vi "sub_load-val.vi"(7 "cmd":enum16{"load", "save"}(ring), 8 "Error in":errorcluster) -> (0 "error out":errorcluster caption="Error out", 3 "config 2":T1={"Ch"="cDAQ1Mod1/ao0", "Max V"=5.0, "Min V"=-5.0, " Rate"=1000.0, "N pts"=100, "sample mode"=10178} {"sample mode" items=["유한 샘플"=10178, "연속 샘플"=10123, "하드웨어 타이밍에 의한 단일 포인트"=12522]})   [LabVIEW 2019]
uses:
  _ctrl/cDAQ-9269 Config.ctl
  _ctrl/TestType.ctl
  _ctrl/rw.ctl
  _ctrl/DL950_config.ctl
  _ctrl/BP4610_config.ctl
  _ctrl/DSP_config.ctl
  Devices/NI Board/cDAQ-9221 AI/Set_NIAI.ctl
  Devices/NI Board/cDAQ-9269 AO/Set_AO_Wave-config.ctl
  Global_params.vi
  Capacitor/Global_params_cap.vi
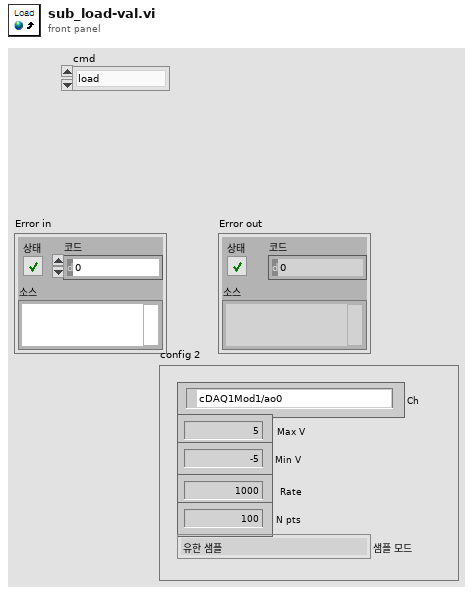
[diagram p1: front panel]
types:
  T1 = typedef "cDAQ-9269 Config.ctl" = cluster{"Ch":tag, "Max V":dbl, "Min V":dbl, " Rate":dbl, "N pts":i32, "sample mode":i32}
  T2 = typedef "TestType.ctl" = enum16{"Manual", "Reg", "Cap", "B1", "B2", "B3"}
  T3 = typedef "rw.ctl" = enum16{"read", "write"}
  T4 = typedef "DL950_config.ctl" = cluster{"Timeout":u32, "Time Div":i32, "Acq Mode":i32, "Record Len":i32, "Record Num":i32, "Start Point":i64, "End Poin":i64, "Visa":refnum<visa-resource-name>, "Config Voltage":cluster{"Enable":bool, "Ch":u16, "V Div":i32, "Coupling":i32, "Probe":i32, "Act.Items":bool, "items":i32[]}[], "Trigger on":bool, "Trigger Level":dbl, "Reset":bool, "Config Temp":cluster{"Channel":u16, "Burn Out":bool, " Type ":i32}[], "Trig Mode":i32, "Trig Pos":dbl, "Trigger Slope":i32, "Trigger Source ":i32, "Trig Start -5":dbl, "End 5":dbl}
  T5 = cluster{"Enable":bool, "Ch":u16, "V Div":i32, "Coupling":i32, "Probe":i32, "Act.Items":bool, "items":i32[]}[]
  T6 = typedef "BP4610_config.ctl" = cluster{"VISA":refnum<visa-resource-name>, "Limit-BP":cluster{"Set":enum16{"Current", "Voltage"}, "Voltage+[V]":dbl, "Current+[A]":dbl, "Voltage-[V]":dbl, "Current-[A]":dbl}, "SET BP":cluster{"Set":enum16{"Current", "Voltage", "FREQ/WAVE"}, "Operation mode":u16, "Voltage[Vp-p]":dbl, "Current[Ap-p]":dbl, "Voltage[V]":dbl, "Current[A]":dbl, "Frequency[Hz]":dbl, "Waveform":enum16{"Sine", "Square", "ARB 1", "ARB 2", "ARB 3", "ARB 4", "ARB 5", "ARB 6", "ARB 7", "ARB 8", "ARB 9", "ARB 10", "ARB 11", "ARB 12", "ARB 13", "ARB 14", "ARB 15", "ARB 16"}}}
  T7 = cluster{"Set":enum16{"Current", "Voltage"}, "Voltage+[V]":dbl, "Current+[A]":dbl, "Voltage-[V]":dbl, "Current-[A]":dbl}
  T8 = typedef "DSP_config.ctl" = cluster{"Port":refnum<visa-resource-name>, "OVP Level":dbl, "OCP Level":dbl, "Current":dbl, "Voltage":dbl}
  T9 = typedef "Set_NIAI.ctl" = cluster{"input terminal":i32, "minimum value":dbl, "maximum value":dbl, "number of samples":i32, "rate":dbl, "sample mode":i32, "physical channels":tag}
  T10 = typedef "Set_AO_Wave-config.ctl" = cluster{"offset":dbl, "Samples":i32, "duty":dbl, "Rate":dbl, "wfm":cluster{"Freq":dbl, "Amp":dbl, "Type":enum16{"Sine Wave", "Triangle Wave", "Square Wave", "Sawtooth Wave"}}}
  T11 = typedef "ref_all.ctl" = cluster{"BP4610 Config":refnum<vi>, "DSP1950 Config":refnum<vi>, "2470-config":refnum<vi>, "cDAQ 9269 AO config":refnum<vi>, "cDAQ 9221 Config":refnum<vi>, "cDAQ-9467 Config":refnum<vi>, "Waveform":refnum<vi>, "DL950 wfm":refnum<vi>, "AI Graph":refnum<vi>, "AO_Wave-config":refnum<vi>, "DL950 items":refnum<vi>, "Volt":refnum<vi>, "Current":refnum<vi>, "AO_Level":refnum<vi>, "RC-Test Judgement ":refnum<vi>, "Log path":refnum<vi>, "시험명":refnum<vi>, "file renew[Hr]":refnum<vi>, "Breakdown-Spec":refnum<vi>, "paste":refnum<vi>, "copy":refnum<vi>, "DL950_config":refnum<vi>, "종료시간":refnum<vi>, "경과시간":refnum<vi>, "Apply":refnum<vi>, "DSP Config LV ":refnum<vi>, "Testconfig":refnum<vi>}
  T12 = typedef "Tpye_ParaAll.ctl" = cluster{"DL950_config":T4, "BP4610 Config":T6, "DSP1950 Config":T8, "DMM 2470 Config":cluster{"Source Mode":enum16{"Voltage", "Current"}, "Source Limit Level":dbl, "Source Level":dbl, "Output_2470":bool}, "cDAQ-9221 Config":T9, "cDAQ-9467 Config":tag, "cDAQ-9269 AO Config":T1, "AO_Wave-config":T10, "DSP1950 Config LV":T8}
  T13 = cluster{"Source Mode":enum16{"Voltage", "Current"}, "Source Limit Level":dbl, "Source Level":dbl, "Output_2470":bool}
  T14 = typedef "cap_config.ctl" = cluster{"Test Mode":T15, "ON time[ms]":dbl, "OFF time[ms]":dbl, "1. 작동시간[분]":dbl, "2. 미작동시간[분]":dbl, "3. 작동시간[분]":dbl, "level[V]":dbl, "duty":dbl, "Freq":dbl, "Voltage+[V]":dbl, "Voltage-[V]":dbl, "Current+[A]":dbl, "Current-[A]":dbl, "출력전압[V]":dbl, "출력전류[A]":dbl, "OVP Level":dbl, "OCP Level":dbl, "Time Div":u16, "Record Len":i32, "방전 기준[V]":dbl, "Repeate (Each Ch)":u32, "Cycle[N]":u32, "작동간격[분]":dbl, "TrigPos[%]":dbl, "시험시간[분]":dbl}
  T15 = typedef "시험모드선택.ctl" = enum16{"6.3.1 온도방치 시험", "6.3.2 저온 작동/방치 시험", "6.3.3 고온 작동/방치 시험", "6.3.4 온도 싸이클 시험", "6.3.6 온습도 싸이클 시험", "6.3.7 고온고습 방치", "6.3.8 결로 시험", "6.3.9 빙결시험", "6.3.11.1 작동가진", "6.3.12 충격시험"}
  T16 = typedef "Breakdown-Spec.ctl" = cluster{"제어단 단선 Irms[mA](이하)":dbl, "제어단 특성 전류 Irms[mA] Max":dbl, "제어단 특성 전류 Irms[mA] Min":dbl, "출력단 단선 Irms[mA](이하)":dbl, "출력단 특성 전류 Irms[mA]  Max":dbl, "출력단 특성전류 Irms[mA]  Min":dbl, "온도[degree]":dbl}
  T17 = typedef "Testing-info.ctl" = cluster{"전체채널수":u8, "현재채널번호":u8, "Irms":dbl, "입력전압":dbl, "입력전류":dbl, "출력전압":dbl, "출력전류":dbl, "온도":dbl, "제어단 단선":bool, "제어단 단락":bool, "제어단 특성변화":bool, "출력단 단선":bool, "출력단 단락":bool, "출력단 특성변화":bool, "출력단 전압":bool, "카운트 일치":bool, "Irms 판정":bool, "온도":bool, "테스트 회수":u32, "TestType":T18, "현재회수":u32, "Ch selection":cluster{"1ch":bool, "2ch":bool, "3ch":bool, "4ch":bool, "5ch":bool, "6ch":bool}, "반복":u32, "Path":path, "파일생성주기":u32, "start time":dbl, "stop time":dbl, "현재반복회수":u32, "NG":cluster{"입출력 카운트":bool, "출력전류RMS":bool}}
  T18 = typedef "sequence_single.ctl" = enum16{"Register", "RC", "B1", "B2", "B3", "Oper_LV", "Oper_HV", "ContR_LV"}
  T19 = typedef "cap_params-all.ctl" = cluster{"Basics":cluster{"TestName":string, "Result path":path, "파일 생성 주기[N]":dbl}, "CapTestConfig":T14, "TestSpec":T16}
  T20 = cluster{"DL950_config":T4, "BP4610 Config":T6, "DSP1950 Config":T8, "DMM 2470 Config":cluster{"Source Mode":enum16{"Voltage", "Current"}, "Source Limit Level":dbl, "Source Level":dbl, "Output_2470":bool}, "cDAQ-9221 Config":T9, "cDAQ-9467 Config":tag, "cDAQ-9269 AO Config":T1, "AO_Wave-config":T10, "Cap Params":T19, "RCconfig":T14}
  T21 = typedef "ref_cap_ctrl-ref.ctl" = cluster{"cDAQ-9467 Config":refnum<vi>, "cDAQ 9221 Config":refnum<vi>, "cDAQ 9269 AO config":refnum<vi>, "AO_Wave-config":refnum<vi>, "TestSpec":refnum<vi>, "DL950_config":refnum<vi>, "BP4610 Config":refnum<vi>, "DSP1950 Config":refnum<vi>, "CapTest":refnum<vi>}
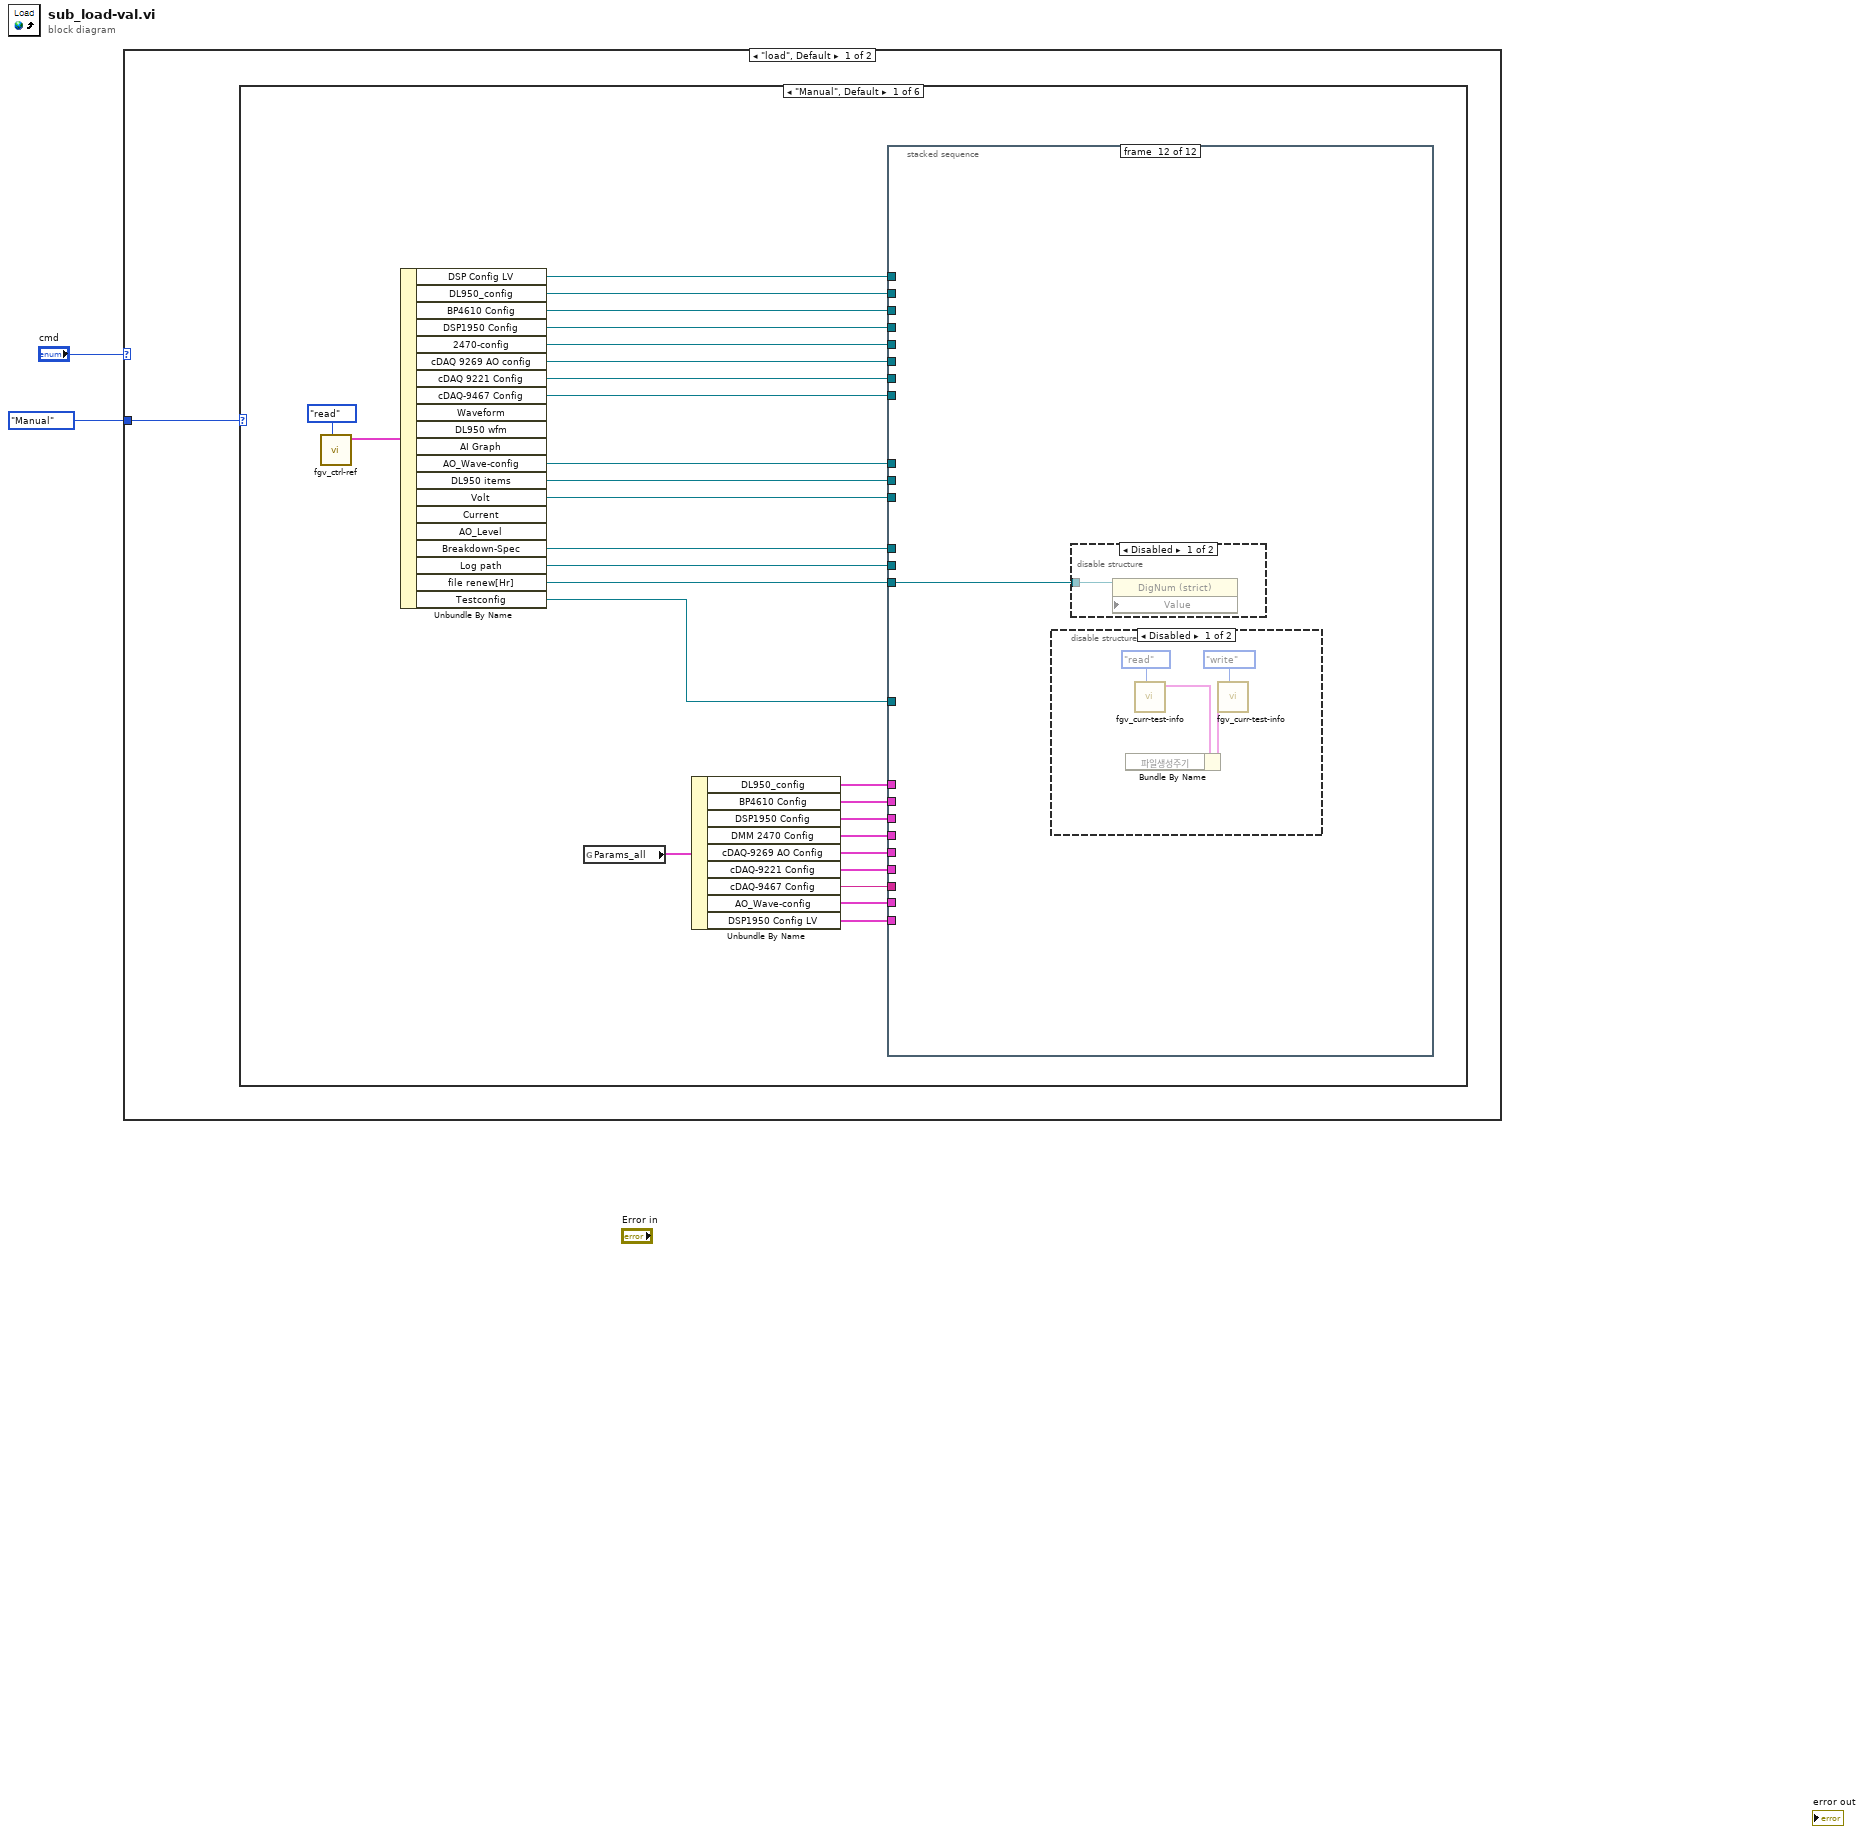
[diagram p0: block diagram]
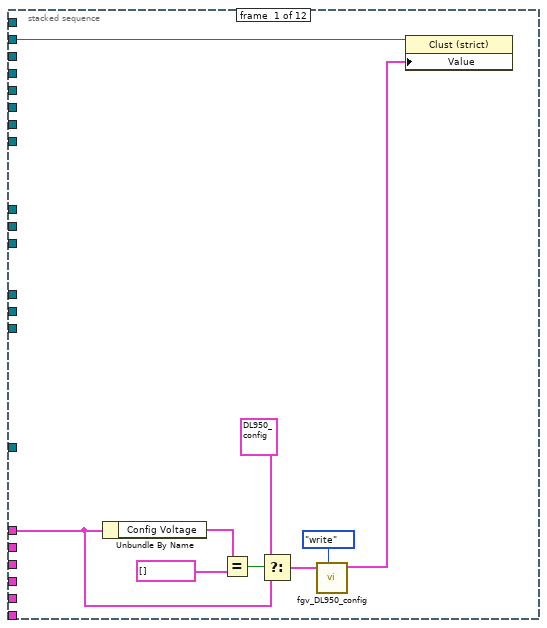
[diagram p2: hidden frame]
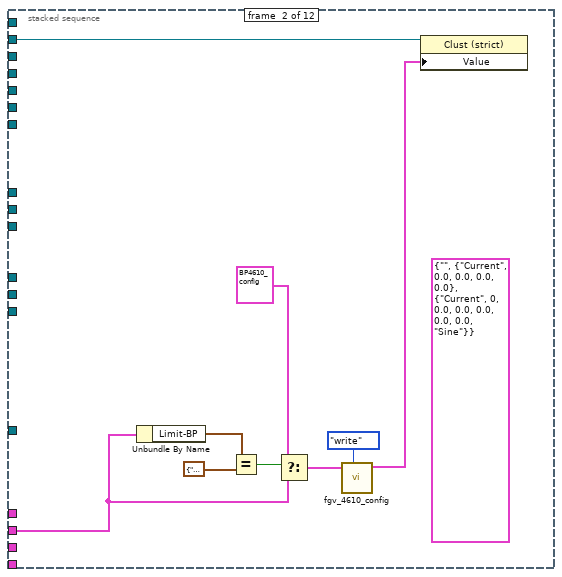
[diagram p3: hidden frame]
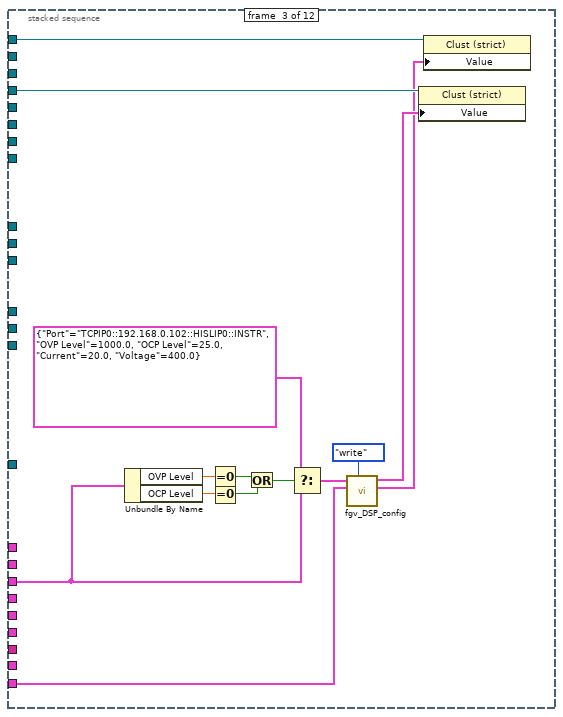
[diagram p4: hidden frame]
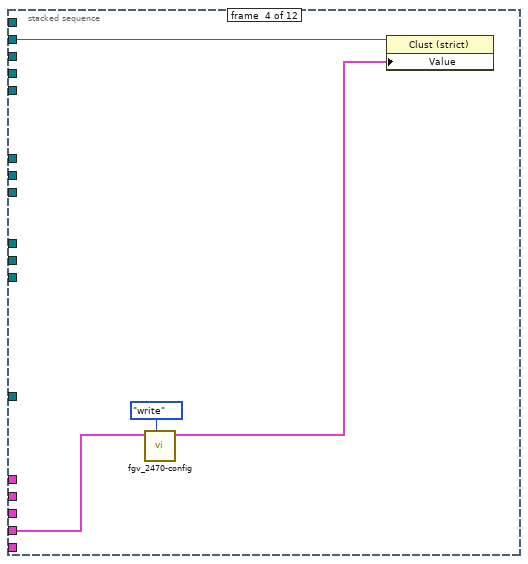
[diagram p5: hidden frame]
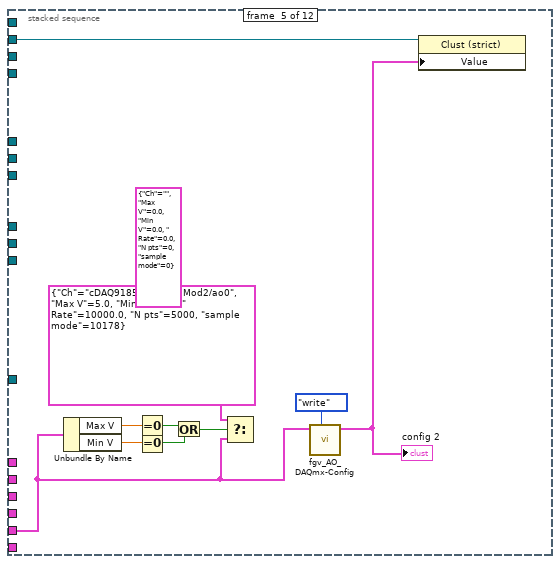
[diagram p6: hidden frame]
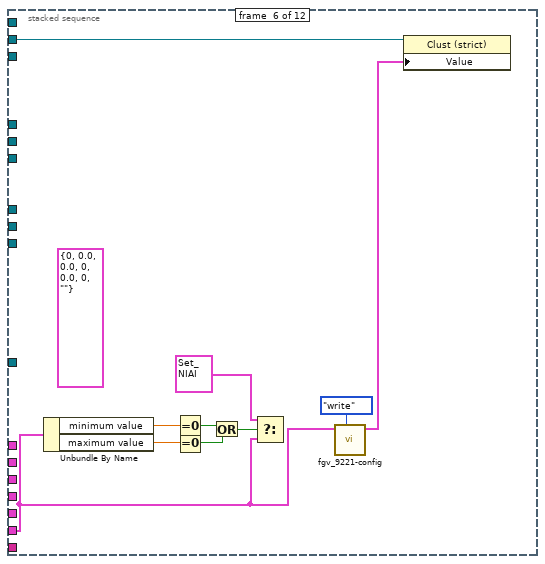
[diagram p7: hidden frame]
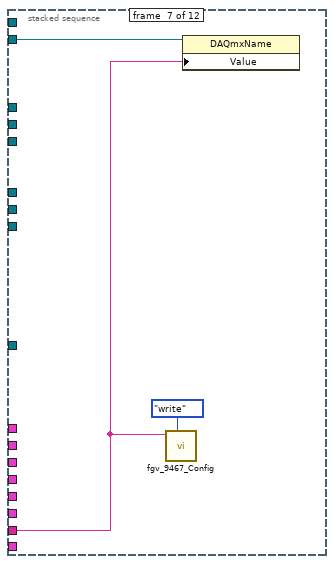
[diagram p8: hidden frame]
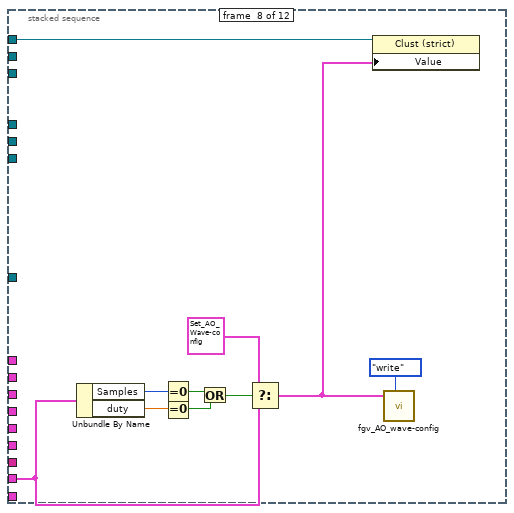
[diagram p9: hidden frame]
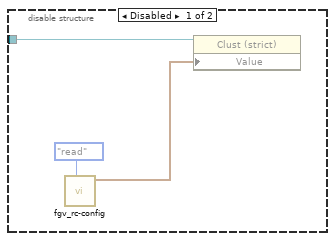
[diagram p11: hidden frame]
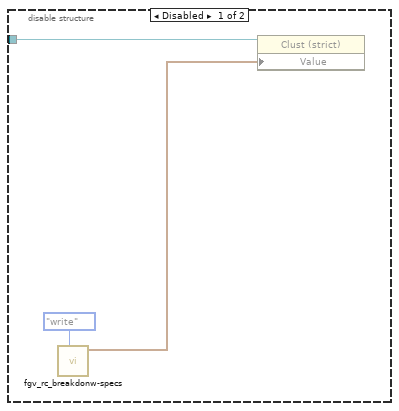
[diagram p13: hidden frame]
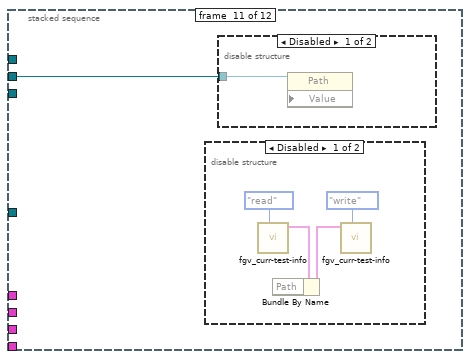
[diagram p14: hidden frame]
diagram:
  n1 = case shown="\"load\", Default" "cmd" {
    tunnel: TestType."Manual" ("TestType") -> [w3 w160]
    frame "load", Default {
      n2 = case shown="\"Manual\", Default" w3 {
        frame "Manual", Default {
          n3 = call "fgv_ctrl-ref.vi"("cmd"=rw."read") -> ("output cluster 2"=w30:T11)  [unwired: 9 in, 1 out]
          n4 = Unbundle By Name(w30) -> ("DSP Config LV"=w5:refnum<vi>, "DL950_config"=w28:refnum<vi>, "BP4610 Config"=w26:refnum<vi>, "DSP1950 Config"=w24:refnum<vi>, "2470-config"=w22:refnum<vi>, "cDAQ 9269 AO config"=w20:refnum<vi>, "cDAQ 9221 Config"=w18:refnum<vi>, "cDAQ-9467 Config"=w16:refnum<vi>, "AO_Wave-config"=w14:refnum<vi>, "DL950 items"=w13:refnum<vi>, "Volt"=w11:refnum<vi>, "Breakdown-Spec"=w9:refnum<vi>, "Log path"=w8:refnum<vi>, "file renew[Hr]"=w7:refnum<vi>, "Testconfig"=w6:refnum<vi>)  [unwired: 5 out]
          n5 = global read "Global_params.vi" "Params_all"() -> (w10:T12)
          n6 = Unbundle By Name(w10) -> ("DL950_config"=w27:T4, "BP4610 Config"=w25:T6, "DSP1950 Config"=w23:T8, "DMM 2470 Config"=w21:T13, "cDAQ-9269 AO Config"=w19:T1, "cDAQ-9221 Config"=w17:T9, "cDAQ-9467 Config"=w15:tag, "AO_Wave-config"=w12:T10, "DSP1950 Config LV"=w4:T8)
          n7 = stacked-sequence {
            tunnel: w28 -> [w38 _ _ _ _ _ _ _ _ _ _ _]
            tunnel: w27 -> [w32 _ _ _ _ _ _ _ _ _ _ _]
            tunnel: w26 -> [_ w48 _ _ _ _ _ _ _ _ _ _]
            tunnel: w25 -> [_ w41 _ _ _ _ _ _ _ _ _ _]
            tunnel: w24 -> [_ _ w62 _ _ _ _ _ _ _ _ _]
            tunnel: w23 -> [_ _ w54 _ _ _ _ _ _ _ _ _]
            tunnel: w22 -> [_ _ _ w66 _ _ _ _ _ _ _ _]
            tunnel: w21 -> [_ _ _ w64 _ _ _ _ _ _ _ _]
            tunnel: w20 -> [_ _ _ _ w76 _ _ _ _ _ _ _]
            tunnel: w19 -> [_ _ _ _ w67 _ _ _ _ _ _ _]
            tunnel: w18 -> [_ _ _ _ _ w86 _ _ _ _ _ _]
            tunnel: w17 -> [_ _ _ _ _ w77 _ _ _ _ _ _]
            tunnel: w16 -> [_ _ _ _ _ _ w89 _ _ _ _ _]
            tunnel: w15 -> [_ _ _ _ _ _ w87 _ _ _ _ _]
            tunnel: w14 -> [_ _ _ _ _ _ _ w99 _ _ _ _]
            tunnel: w13 -> [_ _ _ _ _ _ _ _ _ _ _ _]
            tunnel: w12 -> [_ _ _ _ _ _ _ w91 _ _ _ _]
            tunnel: w11 -> [_ _ _ _ _ _ _ _ _ _ _ _]
            tunnel: w9 -> [_ _ _ _ _ _ _ _ _ w104 _ _]
            tunnel: w8 -> [_ _ _ _ _ _ _ _ _ _ w108 _]
            tunnel: w7 -> [_ _ _ _ _ _ _ _ _ _ _ w114]
            tunnel: w6 -> [_ _ _ _ _ _ _ _ w100 _ _ _]
            tunnel: w5 -> [_ _ w50 _ _ _ _ _ _ _ _ _]
            tunnel: w4 -> [_ _ w51 _ _ _ _ _ _ _ _ _]
            frame #0 {
              n8 = Unbundle By Name(w32) -> ("Config Voltage"=w36:T5)
              n9 = Equal?(x=w36, y=T5 [] ("Config Voltage")) -> (x = y?=w34:bool)
              n10 = Select(t=T4 {"Timeout"=0, "Time Div"=18, "Acq Mode"=0, "Record Len"=4, "Record Num"=0, "Start Point"=0, "End Poin"=60000, "Visa"="TCPIP0::192.168.0.103::inst0::INSTR", "Config Voltage"=[{"Enable"=TRUE, "Ch"=1, "V Div"=15, "Coupling"=1, "Probe"=35, "Act.Items"=FALSE, "items"=[]}, {"Enable"=TRUE, "Ch"=2, "V Div"=23, "Coupling"=1, "Probe"=35, "Act.Items"=FALSE, "items"=[]}, {"Enable"=TRUE, "Ch"=3, "V Div"=23, "Coupling"=1, "Probe"=35, "Act.Items"=FALSE, "items"=[]}, {"Enable"=TRUE, "Ch"=4, "V Div"=23, "Coupling"=1, "Probe"=35, "Act.Items"=FALSE, "items"=[]}, {"Enable"=TRUE, "Ch"=5, "V Div"=6, "Coupling"=1, "Probe"=3, "Act.Items"=FALSE, "items"=[]}, {"Enable"=TRUE, "Ch"=6, "V Div"=15, "Coupling"=1, "Probe"=21, "Act.Items"=FALSE, "items"=[]}], "Trigger on"=TRUE, "Trigger Level"=5.0, "Reset"=FALSE, "Config Temp"=[{"Channel"=9, "Burn Out"=FALSE, " Type "=0}, {"Channel"=10, "Burn Out"=FALSE, " Type "=0}, {"Channel"=11, "Burn Out"=FALSE, " Type "=0}, {"Channel"=12, "Burn Out"=FALSE, " Type "=0}, {"Channel"=13, "Burn Out"=FALSE, " Type "=0}, {"Channel"=14, "Burn Out"=FALSE, " Type "=0}], "Trig Mode"=0, "Trig Pos"=10.0, "Trigger Slope"=0, "Trigger Source "=1, "Trig Start -5"=-5.0, "End 5"=5.0} ("DL950_config 2"), s=w34, f=w32) -> (s? t:f=w33:T4)
              n11 = call "fgv_DL950_config.vi"("cmd"=rw."write", "config"=w33) -> ("config 2"=w37:T4)  [unwired: 8 in, 1 out]
              n12 = property class="Clust (strict)"(reference=w38, "Value"=w37) -> ()  [unwired: 1 in, 2 out]
            }
            frame #1 {
              (unwired) T6 {"VISA"="", "Limit-BP"={"Set"=enum."Current", "Voltage+[V]"=0.0, "Current+[A]"=0.0, "Voltage-[V]"=0.0, "Current-[A]"=0.0}, "SET BP"={"Set"=enum."Current", "Operation mode"=0, "Voltage[Vp-p]"=0.0, "Current[Ap-p]"=0.0, "Voltage[V]"=0.0, "Current[A]"=0.0, "Frequency[Hz]"=0.0, "Waveform"=enum."Sine"}} ("BP4610 Config 2")
              n13 = Unbundle By Name(w41) -> ("Limit-BP"=w45:T7)
              n14 = Equal?(x=w45, y=T7 {"Set"=enum."Current", "Voltage+[V]"=0.0, "Current+[A]"=0.0, "Voltage-[V]"=0.0, "Current-[A]"=0.0} ("Limit-BP")) -> (x = y?=w43:bool)
              n15 = Select(t=T6 {"VISA"="USB0::0x0D4A::0x0040::9426270::INSTR", "Limit-BP"={"Set"=enum."Voltage", "Voltage+[V]"=20.0, "Current+[A]"=5.0, "Voltage-[V]"=-20.0, "Current-[A]"=-5.0}, "SET BP"={"Set"=enum."Voltage", "Operation mode"=1, "Voltage[Vp-p]"=20.0, "Current[Ap-p]"=5.0, "Voltage[V]"=12.0, "Current[A]"=5.0, "Frequency[Hz]"=100.0, "Waveform"=enum."Square"}} ("BP4610 Config 2"), s=w43, f=w41) -> (s? t:f=w42:T6)
              n16 = call "fgv_4610_config.vi"("cmd"=rw."write", "BP4610 Config"=w42) -> ("BP4610 Config 2"=w46:T6)  [unwired: 8 in, 1 out]
              n17 = property class="Clust (strict)"(reference=w48, "Value"=w46) -> ()  [unwired: 1 in, 2 out]
            }
            frame #2 {
              n18 = Unbundle By Name(w54) -> ("OVP Level"=w59:dbl, "OCP Level"=w58:dbl)
              n19 = Equal To 0?(x=w59) -> (x = 0?=w56:bool)
              n20 = Equal To 0?(x=w58) -> (x = 0?=w57:bool)
              n21 = Or(x=w56, y=w57) -> (x .or. y?=w55:bool)
              n22 = Select(t=T8 {"Port"="TCPIP0::192.168.0.102::HISLIP0::INSTR", "OVP Level"=1000.0, "OCP Level"=25.0, "Current"=20.0, "Voltage"=400.0} ("DSP1500 Config 2"), s=w55, f=w54) -> (s? t:f=w53:T8)
              n23 = call "fgv_DSP_config.vi"("cmd"=rw."write", "DSP Config LV IN"=w51, "DSP Config HV IN"=w53) -> ("DSP Config LV OUT"=w49:T8, "DSP Config HV OUT"=w60:T8)  [unwired: 6 in, 1 out]
              n24 = property class="Clust (strict)"(reference=w62, "Value"=w60) -> ()  [unwired: 1 in, 2 out]
              n25 = property class="Clust (strict)"(reference=w50, "Value"=w49) -> ()  [unwired: 1 in, 2 out]
            }
            frame #3 {
              n26 = call "fgv_2470-config.vi"("cmd"=rw."write", "2470-config"=w64) -> ("2470-config 2"=w63:T13)  [unwired: 9 in]
              n27 = property class="Clust (strict)"(reference=w66, "Value"=w63) -> ()  [unwired: 1 in, 2 out]
            }
            frame #4 {
              (unwired) T1 {"Ch"="", "Max V"=0.0, "Min V"=0.0, " Rate"=0.0, "N pts"=0, "sample mode"=0} ("cDAQ 9269 AO config 2")
              n28 = Unbundle By Name(w67) -> ("Max V"=w71:dbl, "Min V"=w70:dbl)
              n29 = Equal To 0?(x=w71) -> (x = 0?=w72:bool)
              n30 = Equal To 0?(x=w70) -> (x = 0?=w73:bool)
              n31 = Or(x=w72, y=w73) -> (x .or. y?=w69:bool)
              n32 = Select(t=T1 {"Ch"="cDAQ9185-213AA55Mod2/ao0", "Max V"=5.0, "Min V"=-5.0, " Rate"=10000.0, "N pts"=5000, "sample mode"=10178} ("cDAQ 9269 AO config 2"), s=w69, f=w67) -> ()  [unwired: 1 out]
              n33 = call "fgv_AO_DAQmx-Config.vi"("cmd"=rw."write", "9269 AO Config"=w67) -> ("config 2"=w74:T1)  [unwired: 8 in, 1 out]
              "config 2" <- w74
              n34 = property class="Clust (strict)"(reference=w76, "Value"=w74) -> ()  [unwired: 1 in, 2 out]
            }
            frame #5 {
              (unwired) T9 {"input terminal"=0, "minimum value"=0.0, "maximum value"=0.0, "number of samples"=0, "rate"=0.0, "sample mode"=0, "physical channels"=""} ("cDAQ 9221 Config 2")
              n35 = Unbundle By Name(w77) -> ("minimum value"=w82:dbl, "maximum value"=w81:dbl)
              n36 = Equal To 0?(x=w82) -> (x = 0?=w83:bool)
              n37 = Equal To 0?(x=w81) -> (x = 0?=w84:bool)
              n38 = Or(x=w83, y=w84) -> (x .or. y?=w80:bool)
              n39 = Select(t=T9 {"input terminal"=10083, "minimum value"=-60.0, "maximum value"=60.0, "number of samples"=1000, "rate"=10000.0, "sample mode"=10123, "physical channels"="cDAQ9185-213AA55Mod3/ai0:7"} ("cDAQ 9221 Config 2"), s=w80, f=w77) -> ()  [unwired: 1 out]
              n40 = call "fgv_9221-config.vi"("cmd"=rw."write", "cDAQ 9221 Config"=w77) -> ("cDAQ 9221 Config 2"=w78:T9)  [unwired: 8 in, 1 out]
              n41 = property class="Clust (strict)"(reference=w86, "Value"=w78) -> ()  [unwired: 1 in, 2 out]
            }
            frame #6 {
              n42 = call "fgv_9467_Config.vi"("cmd"=rw."write", "cDAQ-9467 Config"=w87) -> ()  [unwired: 9 in, 1 out]
              n43 = property class="DAQmxName"(reference=w89, "Value"=w87) -> ()  [unwired: 1 in, 2 out]
            }
            frame #7 {
              n44 = Unbundle By Name(w91) -> ("Samples"=w95:i32, "duty"=w94:dbl)
              n45 = Equal To 0?(x=w95) -> (x = 0?=w96:bool)
              n46 = Equal To 0?(x=w94) -> (x = 0?=w97:bool)
              n47 = Or(x=w96, y=w97) -> (x .or. y?=w93:bool)
              n48 = Select(t=T10 {"offset"=6.0, "Samples"=10000, "duty"=50.0, "Rate"=10000.0, "wfm"={"Freq"=50.0, "Amp"=6.0, "Type"=enum."Square Wave"}} ("AO_Wave-config"), s=w93, f=w91) -> (s? t:f=w92:T10)
              n49 = property class="Clust (strict)"(reference=w99, "Value"=w92) -> ()  [unwired: 1 in, 2 out]
              n50 = call "fgv_AO_wave-config.vi"("cmd"=rw."write", "Square Wave"=w92) -> ()  [unwired: 8 in, 2 out]
            }
            frame #8 {
              n51 = disable-structure shown="Enabled" {
                disable-tunnel: w100 -> [w101 _]
                frame Disabled {
                  n52 = call "fgv_rc-config.vi"("cmd"=rw."read") -> ("Testconfig out"=w102:T14)  [unwired: 9 in, 1 out]
                  n53 = property class="Clust (strict)"(reference=w101, "Value"=w102) -> ()  [unwired: 1 in, 2 out]
                }
                frame Enabled {
                }
              }
            }
            frame #9 {
              n54 = disable-structure shown="Enabled" {
                disable-tunnel: w104 -> [w105 _]
                frame Disabled {
                  n55 = call "fgv_rc_breakdonw-specs.vi"("cmd"=rw."write") -> ("BreakdownSpec 2"=w106:T16)  [unwired: 10 in]
                  n56 = property class="Clust (strict)"(reference=w105, "Value"=w106) -> ()  [unwired: 1 in, 2 out]
                }
                frame Enabled {
                }
              }
            }
            frame #10 {
              n57 = disable-structure shown="Disabled" {
                frame Disabled {
                  n58 = call "fgv_curr-test-info.vi"("cmd"=rw."read") -> ("현재테스트 정보 2"=w113:T17)  [unwired: 10 in]
                  n59 = Bundle By Name(cluster=w113) -> (w112:T17)  [unwired: 1 in]
                  n60 = call "fgv_curr-test-info.vi"("cmd"=rw."write", "현재테스트 정보"=w112) -> ()  [unwired: 9 in, 1 out]
                }
                frame Enabled {
                }
              }
              n61 = disable-structure shown="Disabled" {
                disable-tunnel: w108 -> [w109 _]
                frame Disabled {
                  n62 = property class="Path" props=["Value"](reference=w109) -> ()  [unwired: 2 in, 2 out]
                }
                frame Enabled {
                }
              }
            }
            frame #11 {
              n63 = disable-structure shown="Disabled" {
                frame Disabled {
                  n64 = call "fgv_curr-test-info.vi"("cmd"=rw."read") -> ("현재테스트 정보 2"=w117:T17)  [unwired: 10 in]
                  n65 = Bundle By Name(cluster=w117) -> (w116:T17)  [unwired: 1 in]
                  n66 = call "fgv_curr-test-info.vi"("cmd"=rw."write", "현재테스트 정보"=w116) -> ()  [unwired: 9 in, 1 out]
                }
                frame Enabled {
                }
              }
              n67 = disable-structure shown="Disabled" {
                disable-tunnel: w114 -> [w115 _]
                frame Disabled {
                  n68 = property class="DigNum (strict)" props=["Value"](reference=w115) -> ()  [unwired: 2 in, 2 out]
                }
                frame Enabled {
                }
              }
            }
          }
        }
        frame "Reg" {
        }
        frame "Cap" {
          n69 = disable-structure shown="Enabled" {
            frame Disabled {
              n70 = global read "Global_params_cap.vi" "Params_cap-all"() -> (w138:T20)
              n71 = call "fgv_cap_ctrl-ref.vi"("cmd"=rw."read") -> ("input cluster 2"=w136:T21)  [unwired: 10 in]
              n72 = Unbundle By Name(w138) -> ("Cap Params.CapTestConfig"=w129:T14, "DL950_config"=w121:T4, "BP4610 Config"=w122:T6, "DSP1950 Config"=w123:T8, "DMM 2470 Config"=w124:T13, "cDAQ-9221 Config"=w125:T9, "cDAQ-9467 Config"=w126:tag, "cDAQ-9269 AO Config"=w127:T1, "AO_Wave-config"=w128:T10, "Cap Params.TestSpec"=w120:T16)
              n73 = Unbundle By Name(w136) -> ("CapTest"=w135:refnum<vi>, "cDAQ-9467 Config"=w134:refnum<vi>, "cDAQ 9221 Config"=w133:refnum<vi>, "cDAQ 9269 AO config"=w132:refnum<vi>, "AO_Wave-config"=w131:refnum<vi>, "TestSpec"=w130:refnum<vi>)
              n74 = stacked-sequence {
                tunnel: w135 -> [w140 _ _ _ _ _]
                tunnel: w134 -> [_ w146 _ _ _ _]
                tunnel: w133 -> [_ _ w148 _ _ _]
                tunnel: w132 -> [_ _ _ w152 _ _]
                tunnel: w131 -> [_ _ _ _ w154 _]
                tunnel: w130 -> [_ _ _ _ _ w158]
                tunnel: w129 -> [w139 _ _ _ _ _]
                tunnel: w128 -> [_ _ _ _ w153 _]
                tunnel: w127 -> [_ _ _ w150 _ _]
                tunnel: w126 -> [_ w142 _ _ _ _]
                tunnel: w125 -> [_ _ w147 _ _ _]
                tunnel: w124 -> [_ _ _ _ _ _]
                tunnel: w123 -> [_ _ _ _ _ _]
                tunnel: w122 -> [_ _ _ _ _ _]
                tunnel: w121 -> [_ _ _ _ _ _]
                tunnel: w120 -> [_ _ _ _ _ w156]
                frame #0 {
                  n75 = property class="Clust (strict)"(reference=w140, "Value"=w139) -> ()  [unwired: 1 in, 2 out]
                  n76 = call "fgv_rc-config.vi"("cmd"=rw."write", "Testconfig"=w139) -> ()  [unwired: 8 in, 2 out]
                }
                frame #1 {
                  n77 = property class="DAQmxName"(reference=w146, "Value"=w142) -> ()  [unwired: 1 in, 2 out]
                  n78 = Concatenate Strings(w142, "/line0:31" ("string")) -> (w143:string)
                  n79 = call "fgv_9467_Config.vi"("cmd"=rw."write", "cDAQ-9467 Config"=w143) -> ()  [unwired: 9 in, 1 out]
                }
                frame #2 {
                  n80 = property class="Clust (strict)"(reference=w148, "Value"=w147) -> ()  [unwired: 1 in, 2 out]
                  n81 = call "fgv_9221-config.vi"("cmd"=rw."write", "cDAQ 9221 Config"=w147) -> ()  [unwired: 8 in, 2 out]
                }
                frame #3 {
                  n82 = property class="Clust (strict)"(reference=w152, "Value"=w150) -> ()  [unwired: 1 in, 2 out]
                  n83 = call "fgv_AO_DAQmx-Config.vi"("cmd"=rw."write", "9269 AO Config"=w150) -> ()  [unwired: 8 in, 2 out]
                }
                frame #4 {
                  n84 = property class="Clust (strict)"(reference=w154, "Value"=w153) -> ()  [unwired: 1 in, 2 out]
                  n85 = call "fgv_AO_wave-config.vi"("cmd"=rw."write", "Square Wave"=w153) -> ()  [unwired: 8 in, 2 out]
                }
                frame #5 {
                  n86 = disable-structure shown="Disabled" {
                    disable-tunnel: w158 -> [w159 _]
                    frame Disabled {
                      n87 = property class="Clust (strict)" props=["Value"](reference=w159) -> ()  [unwired: 2 in, 2 out]
                    }
                    frame Enabled {
                    }
                  }
                  n88 = call "fgv_rc_breakdonw-specs.vi"("cmd"=rw."write", "BreakdownSpec"=w156) -> ()  [unwired: 9 in, 1 out]
                }
              }
            }
            frame Enabled {
            }
          }
        }
        frame "B1" {
        }
        frame "B2" {
        }
        frame "B3" {
        }
      }
    }
    frame "save" {
      n89 = case shown="\"Manual\", Default" w160 {
        frame "Manual", Default {
          n90 = call "fgv_ctrl-ref.vi"("cmd"=rw."read") -> ("output cluster 2"=w172:T11)  [unwired: 9 in, 1 out]
          n91 = Unbundle By Name(w172) -> ("cDAQ-9467 Config"=w171:refnum<vi>, "AO_Wave-config"=w169:refnum<vi>, "DL950 items"=w168:refnum<vi>, "Breakdown-Spec"=w164:refnum<vi>, "Log path"=w163:refnum<vi>, "Testconfig"=w162:refnum<vi>)  [unwired: 13 out]
          n92 = stacked-sequence {
            tunnel: [w180 _ _ _ _ _ _ _ _ _] -> w179
            tunnel: [_ w182 _ _ _ _ _ _ _ _] -> w178
            tunnel: [_ _ w185 _ _ _ _ _ _ _] -> w177
            tunnel: [_ _ _ w187 _ _ _ _ _ _] -> w176
            tunnel: [_ _ _ _ w189 _ _ _ _ _] -> w175
            tunnel: [_ _ _ _ _ w191 _ _ _ _] -> w174
            tunnel: w171 -> [_ _ _ _ _ _ w194 _ _ _]
            tunnel: [_ _ _ _ _ _ w193 _ _ _] -> w170
            tunnel: w169 -> [_ _ _ _ _ _ _ _ _ _]
            tunnel: w168 -> [_ _ _ _ _ _ _ _ _ _]
            tunnel: [_ _ _ _ _ _ _ w195 _ _] -> w167
            tunnel: w164 -> [_ _ _ _ _ _ _ _ _ w201]
            tunnel: [_ _ _ _ _ _ _ _ w198 _] -> _
            tunnel: w163 -> [_ _ _ _ _ _ _ _ _ _]
            tunnel: [_ _ _ _ _ _ _ _ _ w202] -> _
            tunnel: w162 -> [_ _ _ _ _ _ _ _ w197 _]
            tunnel: [_ _ w184 _ _ _ _ _ _ _] -> w161
            frame #0 {
              n93 = call "fgv_DL950_config.vi"("cmd"=rw."read") -> ("config 2"=w180:T4)  [unwired: 9 in, 1 out]
            }
            frame #1 {
              n94 = call "fgv_4610_config.vi"("cmd"=rw."read") -> ("BP4610 Config 2"=w182:T6)  [unwired: 9 in, 1 out]
            }
            frame #2 {
              n95 = call "fgv_DSP_config.vi"("cmd"=rw."read") -> ("DSP Config LV OUT"=w184:T8, "DSP Config HV OUT"=w185:T8)  [unwired: 8 in, 1 out]
            }
            frame #3 {
              n96 = call "fgv_2470-config.vi"("cmd"=rw."read") -> ("2470-config 2"=w187:T13)  [unwired: 10 in]
            }
            frame #4 {
              n97 = call "fgv_AO_DAQmx-Config.vi"("cmd"=rw."read") -> ("config 2"=w189:T1)  [unwired: 9 in, 1 out]
            }
            frame #5 {
              n98 = call "fgv_9221-config.vi"("cmd"=rw."read") -> ("cDAQ 9221 Config 2"=w191:T9)  [unwired: 9 in, 1 out]
            }
            frame #6 {
              n99 = property class="DAQmxName"(reference=w194) -> ("Value"=w193:string)  [unwired: 1 in, 2 out]
            }
            frame #7 {
              n100 = call "fgv_AO_wave-config.vi"("cmd"=rw."read") -> ("Square Wave 2"=w195:T10)  [unwired: 9 in, 1 out]
            }
            frame #8 {
              n101 = property class="Clust (strict)"(reference=w197) -> ("Value"=w199:T14)  [unwired: 1 in, 2 out]
              n102 = call "fgv_rc-config.vi"("cmd"=rw."write", "Testconfig"=w199) -> ("Testconfig out"=w198:T14)  [unwired: 8 in, 1 out]
            }
            frame #9 {
              n103 = property class="Clust (strict)"(reference=w201) -> ("Value"=w202:T16)  [unwired: 1 in, 2 out]
            }
          }
          n104 = global read "Global_params.vi" "Params_all"() -> (w166:T12)
          n105 = Bundle By Name(cluster=w166, "DL950_config"=w179, "BP4610 Config"=w178, "DSP1950 Config"=w177, "DMM 2470 Config"=w176, "cDAQ-9269 AO Config"=w175, "cDAQ-9221 Config"=w174, "cDAQ-9467 Config"=w170, "AO_Wave-config"=w167, "DSP1950 Config LV"=w161) -> (w165:T12)
          n106 = global write "Global_params.vi" "Params_all"(w165) -> ()
        }
        frame "Reg" {
        }
        frame "Cap" {
          n107 = call "fgv_cap_ctrl-ref.vi"("cmd"=rw."read") -> ("input cluster 2"=w204:T21)  [unwired: 10 in]
          n108 = Unbundle(w204) -> ("cDAQ-9467 Config"=w203:refnum<vi>)  [unwired: 8 out]
          n109 = stacked-sequence {
            tunnel: [w218 _ _ _ _ _ _ _ _ _] -> w215
            tunnel: [_ w220 _ _ _ _ _ _ _ _] -> w214
            tunnel: [_ _ w222 _ _ _ _ _ _ _] -> w213
            tunnel: [_ _ _ w224 _ _ _ _ _ _] -> w212
            tunnel: [_ _ _ _ w226 _ _ _ _ _] -> w211
            tunnel: [_ _ _ _ _ w228 _ _ _ _] -> w210
            tunnel: w203 -> [_ _ _ _ _ _ w231 _ _ _]
            tunnel: [_ _ _ _ _ _ w230 _ _ _] -> w209
            tunnel: [_ _ _ _ _ _ _ w232 _ _] -> w208
            tunnel: [_ _ _ _ _ _ _ _ w234 _] -> w207
            tunnel: [_ _ _ _ _ _ _ _ _ w236] -> w206
            frame #0 {
              n110 = call "fgv_DL950_config.vi"("cmd"=rw."read") -> ("config 2"=w218:T4)  [unwired: 9 in, 1 out]
            }
            frame #1 {
              n111 = call "fgv_4610_config.vi"("cmd"=rw."read") -> ("BP4610 Config 2"=w220:T6)  [unwired: 9 in, 1 out]
            }
            frame #2 {
              n112 = call "fgv_DSP_config.vi"("cmd"=rw."read") -> ("DSP Config HV OUT"=w222:T8)  [unwired: 8 in, 2 out]
            }
            frame #3 {
              n113 = call "fgv_2470-config.vi"("cmd"=rw."read") -> ("2470-config 2"=w224:T13)  [unwired: 10 in]
            }
            frame #4 {
              n114 = call "fgv_AO_DAQmx-Config.vi"("cmd"=rw."read") -> ("config 2"=w226:T1)  [unwired: 9 in, 1 out]
            }
            frame #5 {
              n115 = call "fgv_9221-config.vi"("cmd"=rw."read") -> ("cDAQ 9221 Config 2"=w228:T9)  [unwired: 9 in, 1 out]
            }
            frame #6 {
              n116 = property class="DAQmxName"(reference=w231) -> ("Value"=w230:string)  [unwired: 1 in, 2 out]
            }
            frame #7 {
              n117 = disable-structure shown="Disabled" {
                disable-tunnel: [w233 _] -> w232
                frame Disabled {
                  n118 = property class="Path"() -> ("Value"=w233:path)  [unwired: 2 in, 2 out]
                }
                frame Enabled {
                }
              }
            }
            frame #8 {
              n119 = disable-structure shown="Disabled" {
                disable-tunnel: [w235 _] -> w234
                frame Disabled {
                  n120 = property class="Str"() -> ("Value"=w235:string)  [unwired: 2 in, 2 out]
                }
                frame Enabled {
                }
              }
            }
            frame #9 {
              n121 = call "fgv_AO_wave-config.vi"("cmd"=rw."read") -> ("Square Wave 2"=w236:T10)  [unwired: 9 in, 1 out]
            }
          }
          n122 = global read "Global_params_cap.vi" "Params_cap-all"() -> (w216:T20)
          n123 = Bundle By Name(cluster=w216, "DL950_config"=w215, "BP4610 Config"=w214, "DSP1950 Config"=w213, "DMM 2470 Config"=w212, "cDAQ-9269 AO Config"=w211, "cDAQ-9221 Config"=w210, "cDAQ-9467 Config"=w209, "Cap Params.Basics.Result path"=w208, "Cap Params.Basics.TestName"=w207, "AO_Wave-config"=w206) -> (w217:T20)
          n124 = global write "Global_params_cap.vi" "Params_cap-all"(w217) -> ()
        }
        frame "B1" {
        }
        frame "B2" {
        }
        frame "B3" {
        }
      }
    }
  }
